vi "One Button Dialog w. Icon.vi"(7 "Window Title (\"\")":string, 8 "Symbol":T1, 10 "button name (OK)":string="OK", 11 "message":string) -> (3 "T":bool=TRUE)   [LabVIEW 2012, in "Workspace MultiY Graph.lvlib" / "Alert Dialogs.lvlib"]
uses:
  Alert Dialogs.lvlib
  Dlg Symbol.ctl
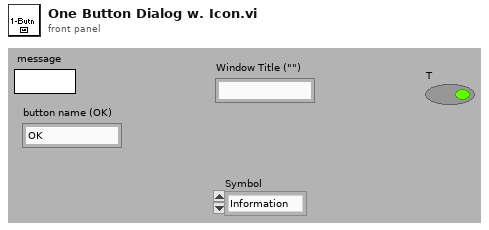
[diagram p1: front panel]
types:
  T1 = typedef "Workspace MultiY Graph.lvlib/Alert Dialogs.lvlib/Dlg Symbol.ctl" = enum16{"Information", "Help", "Warning", "Error"}
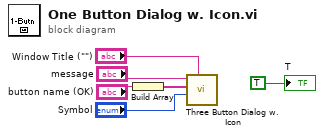
[diagram p0: block diagram]
diagram:
  n1 = Build Array("button name (OK)") -> (w5:string[])
  n2 = call "Three Button Dialog w. Icon.vi"("Window Title (\"\")"="Window Title (\"\")", "Symbol"="Symbol", "Button Strings"=w5, "Message"="message") -> ()  [unwired: 3 in, 5 out]
  "T" <- TRUE
